vi "Get Current Camera.vi"(8 "error in (no error)":errorcluster, 11 "cameraHandle":i32) -> (0 "error out":errorcluster, 2 "function return":u32, 3 "cameraHandle out":i32)   [LabVIEW 2014, in "atmcd32d.lvlib"]
doc: "unsigned int WINAPI GetCurrentCamera(long * cameraHandle);"
uses:
  atmcd32d.lvlib
  atmcd32d.dll
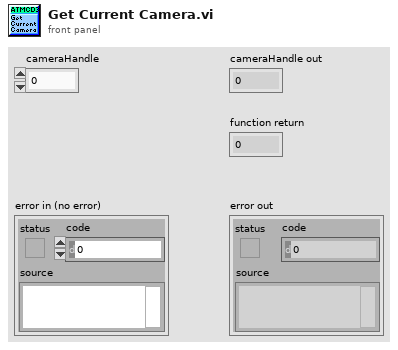
[diagram p1: front panel]
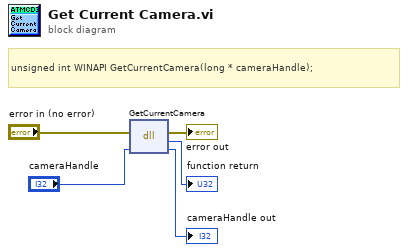
[diagram p0: block diagram]
diagram:
  # "unsigned int WINAPI GetCurrentCamera(long * cameraHandle);"
  n1 = dll-call lib="C:/Users/Bakir/Documents/Lambda2-Testing/lib/Andorlib/atmcd32d.*" fn="GetCurrentCamera"(error in="error in (no error)", "cameraHandle"="cameraHandle") -> (error out=→"error out":errorcluster, →"function return":u32, "cameraHandle"=→"cameraHandle out":i32)  [unwired: 2 in, 1 out]
